vi "LVPortEventGlobals.vi"() -> ()   [LabVIEW 2017]
panel:
  out "EventStreamByID":variant
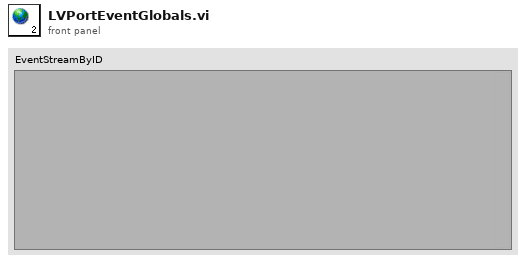
[diagram p1: front panel]
diagram:
